vi "英维克MB_api.vi"(6 "Slave ID":u8=1, 7 "STEP":T1(ring)=enum."read", 8 "Error in":errorcluster caption="Error in (no error)", 9 "values":u16[](array[numeric]), 10 "quantity":u16, 11 "starting address":u16 format="%04xH") -> (0 "error out":errorcluster, 2 "MB session out":refnum<class "MB_Master.lvclass">, 3 "Registers":u16[](array[numeric]))   [LabVIEW 2016, in "环境动力监测库.lvlib" / "空调库.lvlib"]
uses:
  <vilib>/Plasmionique/MB Master/MB_Master/MB_Master.lvclass
  <vilib>/Plasmionique/MB Master/MB_Master_Serial/MB_Master_Serial.lvclass
  C:/Program Files (x86)/National Instruments/LabVIEW 2016/vi.lib/Plasmionique/MB Master/MB_Master/MB_Master.lvclass
  <vilib>/Plasmionique/MB Master/MB_Master_TCP/MB_Master_TCP.lvclass
  <vilib>/Plasmionique/MB Master/MB Master.lvlib
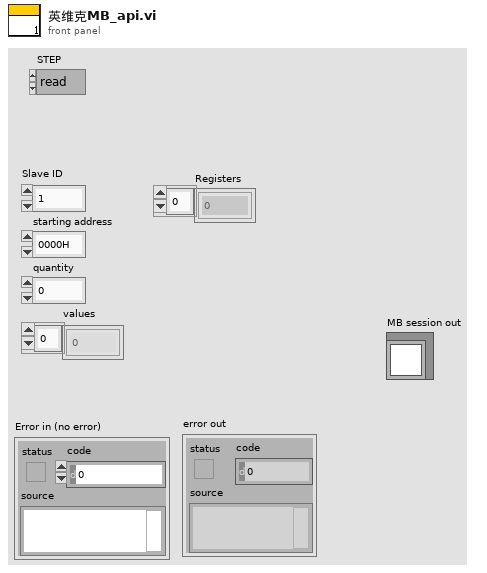
[diagram p1: front panel]
types:
  T1 = enum16{"open", "read", "write single", "write", "close"}
  T2 = cluster{"型号选择":enum16{"黑盾", "英维克", "仁科测控RS-KTC-N01"}, "MB session in":refnum<class "MB_Master.lvclass">, "英维克空调寄存器":u16[], "通讯状态":bool, "PORT":string, "IP":string, "Slave ID ":u8, "Serial Config":cluster{"baud rate (bps)":u32, "stop bits":u16, "parity":u16, "flow control":u16, "timeout":u32, "retries":i32}, "VISA Resource":refnum<visa-resource-name>, "MB通信方式选择":enum16{"串口", "TCP"}, "系统参数":cluster{"空调开启点":u16, "空调灵敏点":u16, "加热开启点":u16, "加热灵敏度":u16, "高温告警点":u16, "低温告警点":u16}}
  T3 = cluster{"baud rate (bps)":u32, "stop bits":u16, "parity":u16, "flow control":u16, "timeout":u32, "retries":i32}
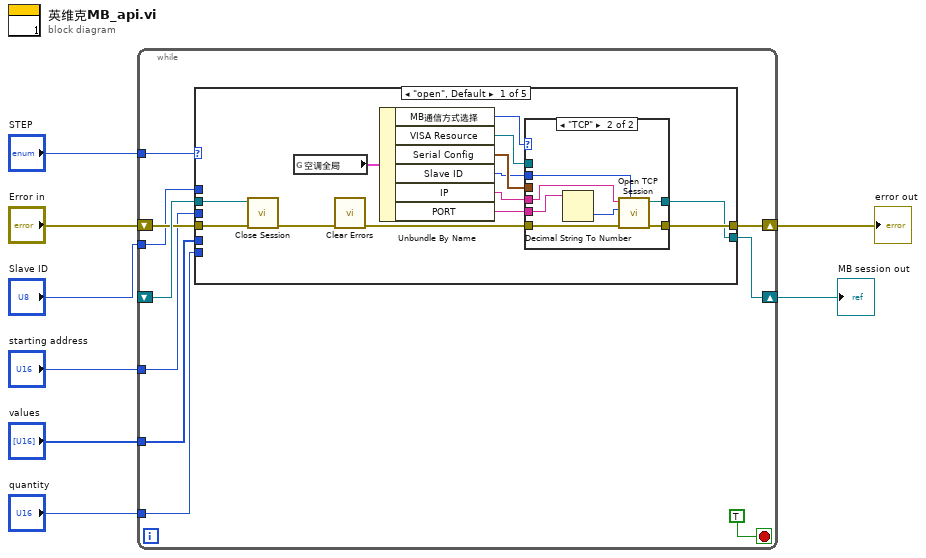
[diagram p0: block diagram]
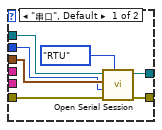
[diagram p2: hidden frame]
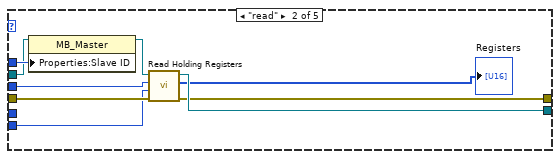
[diagram p3: hidden frame]
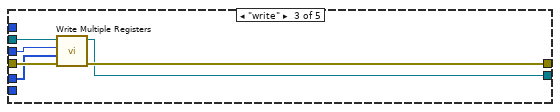
[diagram p4: hidden frame]
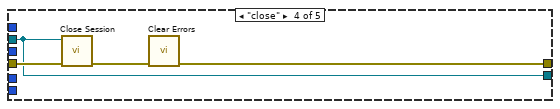
[diagram p5: hidden frame]
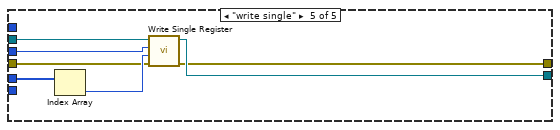
[diagram p6: hidden frame]
diagram:
  n1 = while {
    shift-right: [w10] -> w1
    shift-left: _ -> [w18]
    shift-right: [w9] -> w7
    shift-left: "Error in" -> [w17]
    tunnel: "Slave ID" -> [w16]
    tunnel: "starting address" -> [w15]
    tunnel: "quantity" -> [w14]
    tunnel: "STEP" -> [w13]
    tunnel: "values" -> [w12]
    stop <- TRUE stop-if-true
    n2 = case shown="\"open\", Default" w13 {
      tunnel: w18 -> [w29 w47 w58 w63 w71]
      tunnel: w17 -> [w28 w54 w60 w64 w67]
      tunnel: [w30 w53 w57 w63 w66] -> w10
      tunnel: [w31 w52 w59 w61 w65] -> w9
      tunnel: w16 -> [_ w50 _ _ _]
      tunnel: w15 -> [_ w49 w56 _ w68]
      tunnel: w14 -> [_ w48 _ _ _]
      tunnel: w12 -> [_ _ w55 _ w70]
      frame "open", Default {
        n3 = call-dynamic "Close Session.vi"("error in (no error)"=w28, "MB session in"=w29) -> ("error out"=w27:errorcluster)  [unwired: 9 in]
        n4 = global read "断电保存全局变量.vi" "空调全局"() -> (w25:T2)
        n5 = call <vilib>:"Clear Errors.vi"("error in (no error)"=w27) -> ("error out"=w26:errorcluster)  [unwired: 5 in, 1 out]
        n6 = Unbundle By Name(w25) -> ("MB通信方式选择"=w24:enum16{"串口", "TCP"}, "VISA Resource"=w23:refnum<visa-resource-name>, "Serial Config"=w22:T3, "Slave ID"=w21:u8, "IP"=w20:string, "PORT"=w19:string)
        n7 = case shown="\"TCP\"" w24 {
          tunnel: [w37 w43] -> w31
          tunnel: [w35 w42] -> w30
          tunnel: w26 -> [w36 w44]
          tunnel: w23 -> [w34 _]
          tunnel: w22 -> [w33 _]
          tunnel: w21 -> [w32 w41]
          tunnel: w20 -> [_ w40]
          tunnel: w19 -> [_ w39]
          frame "串口", Default {
            n8 = call <vilib>:"Open Serial Session.vi"("Mode (RTU)"=enum16{"RTU", "ASCII"}."RTU", "Error in"=w36, "Slave ID"=w32, "Serial Config"=w33, "VISA Resource"=w34) -> ("Error out"=w37:errorcluster, "MB_Serial session"=w35:refnum<class "MB_Master_Serial.lvclass">)  [unwired: 5 in]
          }
          frame "TCP" {
            n9 = Decimal String To Number(string=w39) -> (number=w45:i32)  [unwired: 2 in, 1 out]
            n10 = call <vilib>:"Open TCP Session.vi"("Slave ID (255)"=w41, "error in (no error)"=w44, "Port (502)"=w45, "IP Address"=w40) -> ("error out"=w43:errorcluster, "MB_TCP session"=w42:refnum<class "MB_Master_TCP.lvclass">)  [unwired: 6 in]
          }
        }
      }
      frame "read" {
        n11 = property class="MB_Master"(reference=w47, "Properties:Slave ID"=w50) -> (reference out=w46:refnum<class "MB_Master.lvclass">)  [unwired: 1 in, 1 out]
        n12 = call <vilib>:"Read Holding Registers.vi"("error in (no error)"=w54, "quantity"=w48, "starting address"=w49, "MB session in"=w46) -> ("error out"=w52:errorcluster, "Registers"=→"Registers":u16[], "MB session out"=w53:refnum<class "MB_Master.lvclass">)  [unwired: 5 in]
      }
      frame "write" {
        n13 = call <vilib>:"Write Multiple Registers.vi"("error in (no error)"=w60, "values"=w55, "starting address"=w56, "MB session in"=w58) -> ("error out"=w59:errorcluster, "MB session out"=w57:refnum<class "MB_Master.lvclass">)  [unwired: 6 in]
      }
      frame "close" {
        n14 = call-dynamic "Close Session.vi"("error in (no error)"=w64, "MB session in"=w63) -> ("error out"=w62:errorcluster)  [unwired: 9 in]
        n15 = call <vilib>:"Clear Errors.vi"("error in (no error)"=w62) -> ("error out"=w61:errorcluster)  [unwired: 5 in, 1 out]
      }
      frame "write single" {
        n16 = Index Array(array=w70) -> (element=w69:u16)  [unwired: 1 in]
        n17 = call <vilib>:"Write Single Register.vi"("error in (no error)"=w67, "value"=w69, "address"=w68, "MB session in"=w71) -> ("error out"=w65:errorcluster, "MB session out"=w66:refnum<class "MB_Master.lvclass">)  [unwired: 6 in]
      }
    }
  }
  "error out" <- w7
  "MB session out" <- w1
